vi "TDMS2TDMWriteLogFile.vi"(8 "error in (no error)":errorcluster, 11 "Log File Path":path) -> (0 "error out":errorcluster)   [LabVIEW 2017]
doc: "This VI writes the log text to file."
uses:
  <vilib>/Utility/tdmsutil.llb/TDMS2TDMLogOperation.ctl
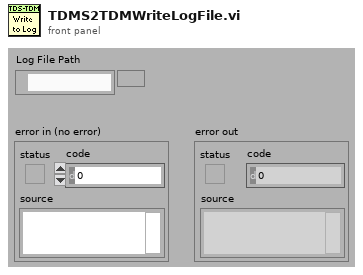
[diagram p1: front panel]
types:
  T1 = typedef "TDMS2TDMLogOperation.ctl" = enum16{"Initialize", "Data Conversion", "Name Conversion", "Write Log File"}
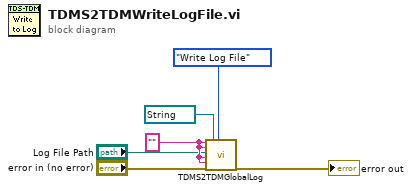
[diagram p0: block diagram]
diagram:
  w4 = "" ("Original Name")
  n1 = call <vilib>:"TDMS2TDMGlobalLog.vi"("Original Name"=w4, "New Name"=w4, "Log File Path"="Log File Path", "Original Datatype"=w4, "New Datatype"=w4, "error in (no error)"="error in (no error)", "Str Refnum"=refnum<vi> refnum, "Operation"=TDMS2TDMLogOperation."Write Log File") -> ("error out"=→"error out":errorcluster)  [unwired: 11 in]
